vi "randomGen.vi"(10 "dzielnikMapy":T1, 11 "Wielkosc mapy":T1) -> (3 "wygenerowane współrzędne":cluster{u64, u64})   [LabVIEW 2020]
uses:
  <vilib>/Utility/miscctls.llb/LVBoundsTypeDef.ctl
  <vilib>/numeric/Random Number (Range) U64.vi
  <vilib>/numeric/sub_Random U32.vi
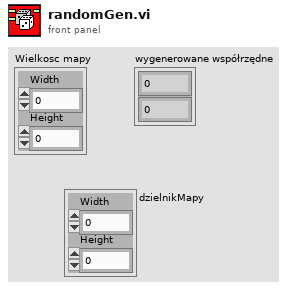
[diagram p1: front panel]
types:
  T1 = typedef "LVBoundsTypeDef.ctl" = cluster{"Width":u32, "Height":u32}
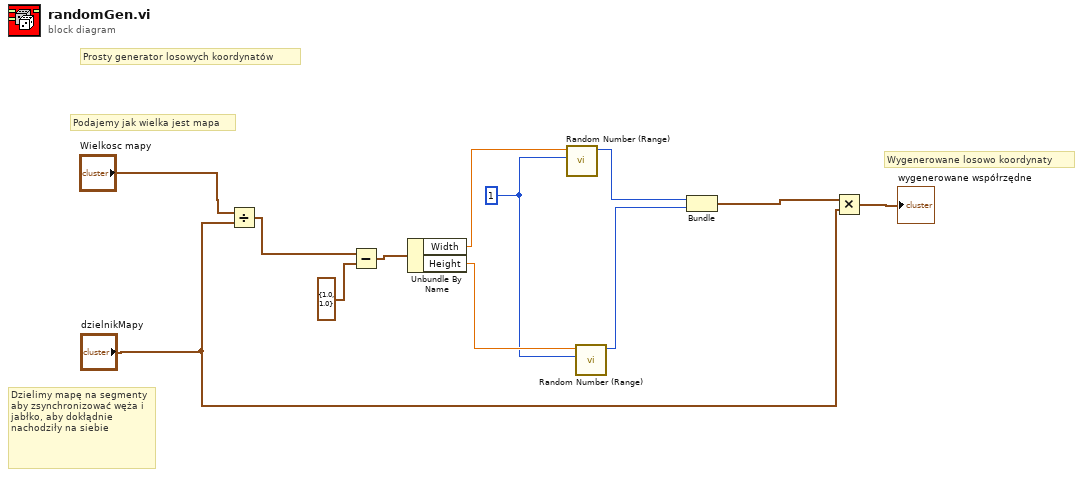
[diagram p0: block diagram]
diagram:
  w6 = u64 1 ("lower bound (0)")
  # "Wygenerowane losowo koordynaty"
  # "Dzielimy mapę na segmenty aby zsynchronizować węża i jabłko, aby dokłądnie nachodziły na siebie"
  # "Podajemy jak wielka jest mapa"
  # "Prosty generator losowych koordynatów"
  n1 = Divide(x="Wielkosc mapy", y="dzielnikMapy") -> (x/y=w3:cluster{"Width":dbl, "Height":dbl})
  n2 = Subtract(x=w3, y=cluster{"Width":dbl, "Height":dbl} {"Width"=1.0, "Height"=1.0}) -> (x-y=w2:cluster{"Width":dbl, "Height":dbl})
  n3 = Unbundle By Name(w2) -> ("Width"=w8:dbl, "Height"=w7:dbl)
  n4 = call-poly <vilib>:"Random Number (Range).vi"("lower bound (0)"=w6, "upper bound (100)"=w8) -> ("number"=w9:u64)  [unwired: 9 in]
  n5 = call-poly <vilib>:"Random Number (Range).vi"("lower bound (0)"=w6, "upper bound (100)"=w7) -> ("number"=w10:u64)  [unwired: 9 in]
  n6 = Bundle("number"=w9, "number"=w10) -> (w11:cluster{"number":u64, "number":u64})  [unwired: 1 in]
  n7 = Multiply(x=w11, y="dzielnikMapy") -> (x*y=→"wygenerowane współrzędne":cluster{u64, u64})
